vi "Numeric Control - Slide.vi"() -> ()   [LabVIEW 2013]
doc: "Sample numeric display item."
uses:
  <vilib>/NI Veristand/Display Template Support/Display Template Support.llb/cluster_Screen Item Settings.ctl
  <vilib>/NI Veristand/Display Template Support/Display Template Support.llb/cluster_Graph Scale Settings.ctl
  <vilib>/NI Veristand/Display Template Support/Display Template Support.llb/cluster_Graph Plot Settings.ctl
  <vilib>/NI Veristand/Display Template Support/Display Template Support.llb/cluster_Graph Handler Message.ctl
  <vilib>/NI Veristand/Display Template Support/Display Template Support.llb/enum_Graph Handler Message.ctl
panel:
  in  "Item.Data":T1
  in  "Numeric Control":dbl(slide) scale=0.0..20.0
  out "Label":string="Numeric"
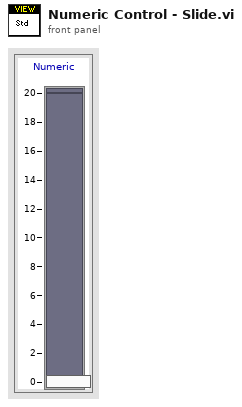
[diagram p1: front panel]
types:
  T1 = typedef "cluster_Screen Item Settings.ctl" = cluster{"Template VI":string, "Position X":i32, "Position Y":i32, "Custom":string, "Show Title Bar":bool, "ID":i32, "Always On Top":bool, "Allow Resize":bool, "Allow Minimize":bool, "Allow Close":bool, "Size to Screen":bool, "Screen.ID":i32, "State":enum16{"Normal", "New"}, "Title":string, "Window Bounds":cluster{"[0]":i16, "[1]":i16, "[2]":i16, "[3]":i16}, "Channel Ref":u64, "Unit":string, "Default Units?":bool, "Flash Limit?":bool, "Color 1":u32, "Color 2":u32, "Color 3":u32, "Color 4":u32, "Bck Color":u32, "Fore Color":u32, "Limit 1":dbl, "Limit 2":dbl, "Limit 3":dbl, "Limit 4":dbl, "Limit Mode 1":i32, "Limit Mode 2":i32, "Limit Mode 3":i32, "Limit Mode 4":i32, "Scale Precision":i32, "Scale Min":dbl, "Scale Max":dbl, "Format":i32, "Precision":i32, "Background Type":i32, "IDs":i32[], "Units":string[], "Labels":string[], "Scale Factor":dbl, "Scale Offset":dbl, "YScale Index":u32[], "XScale":T2, "YScales":T2[], "Plots":T3[], "Update Period":dbl, "History Length":dbl, "My.Ref":refnum<vi>, "Is Control?":bool, "Channel Paths":string[], "Custom Data":variant}
  T2 = typedef "cluster_Graph Scale Settings.ctl" = cluster{"Format":u8, "Precision":u8, "Fit":u8, "Label":string, "Use Default Label":bool, "Label Visible":bool, "Min":dbl, "Max":dbl}
  T3 = typedef "cluster_Graph Plot Settings.ctl" = cluster{"Bar Style":u8, "Fill To":i16, "Fill/PtColor":u32, "Line Style":u8, "Line Width":u8, "Color":u32, "Interp":u8, "Point Style":u8}
  T4 = typedef "cluster_Graph Handler Message.ctl" = cluster{"Message":T5, "Data":variant}
  T5 = typedef "enum_Graph Handler Message.ctl" = enum16{"None", "Stop", "Hold", "Update Channels", "New Settings", "Control Value", "Edit Value"}
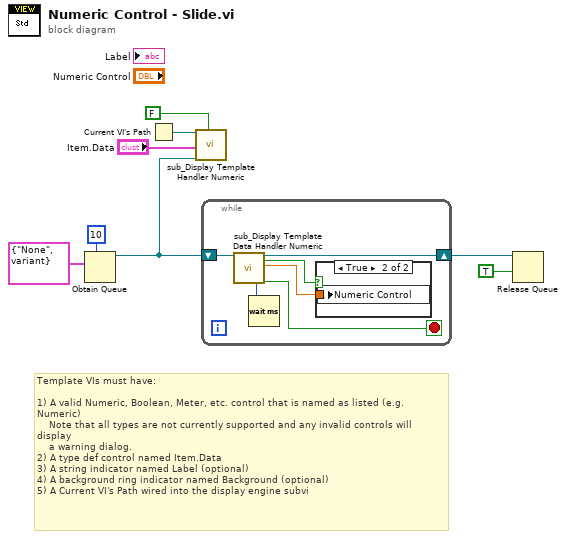
[diagram p0: block diagram]
diagram:
  # "Template VIs must have:\n\n1) A valid Numeric, Boolean, Meter, etc. control that is named as listed (e.g. Numeric)\n    Note that all types are not currently supported and any invalid controls will display\n    a warning dialog.\n2) A type def control named Item.Data\n3) A string indicator named Label (optional)\n4) A background ring indicator named Background (optional)\n5) A Current VI's Path wired into the display engine subvi"
  n1 = Obtain Queue(max queue size (-1, unlimited)=10, element data type=T4 {"Message"=enum."None", "Data"=variant} ("Message")) -> (queue out=w2:refnum<queue>)  [unwired: 2 in, 3 out]
  n2 = Current VI's Path() -> (path=w8:path)
  n3 = call <vilib>:"sub_Display Template Handler Numeric.vi"("Parent.Path"=w8, "Item.Data"="Item.Data", "queue"=w2, "Use Transparency?"=FALSE) -> ()  [unwired: 16 out]
  n4 = while {
    shift-right: [w14] -> w6
    shift-left: w2 -> [w13]
    stop <- w11 stop-if-true
    n5 = call <vilib>:"sub_Display Template Data Handler Numeric.vi"("queue"=w13) -> ("Wait.Time"=w12:u32, "queue out"=w14:refnum<queue>, "Update.Value"=w9:bool, "Numeric.Value"=w10:dbl, "Stop"=w11:bool)  [unwired: 14 out]
    n6 = Wait (ms)(milliseconds to wait=w12) -> ()  [unwired: 1 out]
    n7 = case shown="True" w9 {
      tunnel: w10 -> [_ w15]
      frame False {
      }
      frame True {
        n8 = local write "Numeric Control"(w15) -> ()
      }
    }
  }
  n9 = Release Queue(queue=w6, force destroy? (F)=TRUE) -> ()  [unwired: 1 in, 3 out]
